vi "Temperature Degree to analog Value  (SubVI).vi"(11 "Temperature (C)":dbl) -> (3 "Temperature Analog Value":u8)   [LabVIEW 2024]
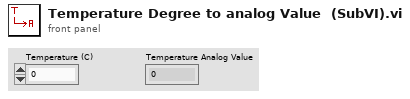
[diagram p1: front panel]
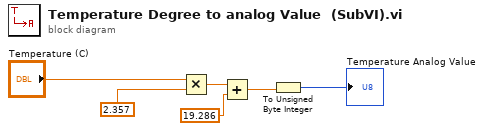
[diagram p0: block diagram]
diagram:
  n1 = Multiply(x="Temperature (C)", y=2.357) -> (x*y=w3:dbl)
  n2 = Add(x=w3, y=19.286) -> (x+y=w5:dbl)
  n3 = To Unsigned Byte Integer(number=w5) -> (unsigned 8bit integer=→"Temperature Analog Value":u8)
